vi "CheckLatinAlfabet.vi"(0 "str":string, 11 "error in (no error)":errorcluster) -> (6 "OK":bool, 15 "error out":errorcluster)   [LabVIEW 2019]
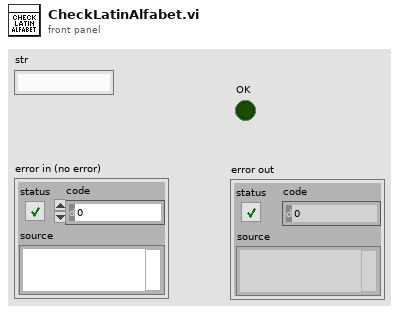
[diagram p1: front panel]
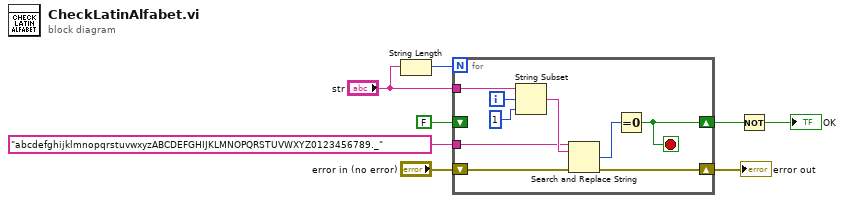
[diagram p0: block diagram]
diagram:
  n1 = String Length(string="str") -> (length=w8:i32)
  n2 = for {
    N: w8 -> [_]
    tunnel: "str" -> [w17]
    tunnel: "abcdefghijklmnopqrstuvwxyzABCDEFGHIJKLMNOPQRSTUVWXYZ0123456789._" -> [w13]
    shift-right: [w11] -> w4
    shift-left: "error in (no error)" -> [w12]
    shift-right: [w9] -> w3
    shift-left: FALSE -> [_]
    i -> [w16]
    stop <- w9 stop-if-true
    n3 = String Subset(string=w17, offset (0)=w16, length (rest)=1 ("length (rest)")) -> (substring=w14:string)
    n4 = Search and Replace String(input string=w13, search string=w14, error in=w12) -> (number of replacements=w10:i32, error out=w11:errorcluster)  [unwired: 5 in, 2 out]
    n5 = Equal To 0?(x=w10) -> (x = 0?=w9:bool)
  }
  "error out" <- w4
  n6 = Not(x=w3) -> (.not. x?=→"OK":bool)
